vi "movimentacao basica.vi"() -> ()   [LabVIEW 2020]
uses:
  <vilib>/Utility/inputDevices.llb/joystickAcquire.vi
  <vilib>/Utility/inputDevices.llb/closeJoystick.vi
panel:
  out "Motor Esquerda":dbl
  out "Motor Direita":dbl
  out "Acelerando Trás":bool
  out "Acelerando Frente":bool
  out "Trás":bool
  out "Frente":bool
  out "joystick info":T1(array[cluster])
  out "axis info":T2
  out "button info":T3
  out "direction info":T4
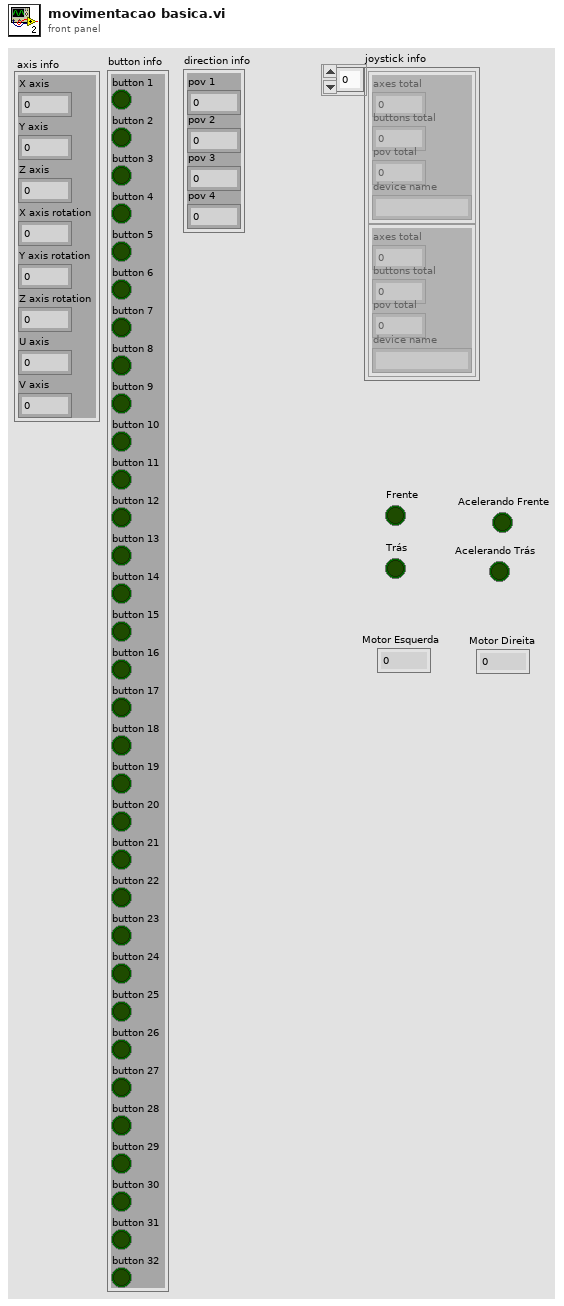
[diagram p1: front panel]
types:
  T1 = cluster{"axes total":u32, "buttons total":u32, "pov total":u32, "device name":string}[]
  T2 = cluster{"X axis":i32, "Y axis":i32, "Z axis":i32, "X axis rotation":i32, "Y axis rotation":i32, "Z axis rotation":i32, "U axis":i32, "V axis":i32}
  T3 = cluster{"button 1":bool, "button 2":bool, "button 3":bool, "button 4":bool, "button 5":bool, "button 6":bool, "button 7":bool, "button 8":bool, "button 9":bool, "button 10":bool, "button 11":bool, "button 12":bool, "button 13":bool, "button 14":bool, "button 15":bool, "button 16":bool, "button 17":bool, "button 18":bool, "button 19":bool, "button 20":bool, "button 21":bool, "button 22":bool, "button 23":bool, "button 24":bool, "button 25":bool, "button 26":bool, "button 27":bool, "button 28":bool, "button 29":bool, "button 30":bool, "button 31":bool, "button 32":bool}
  T4 = cluster{"pov 1":i32, "pov 2":i32, "pov 3":i32, "pov 4":i32}
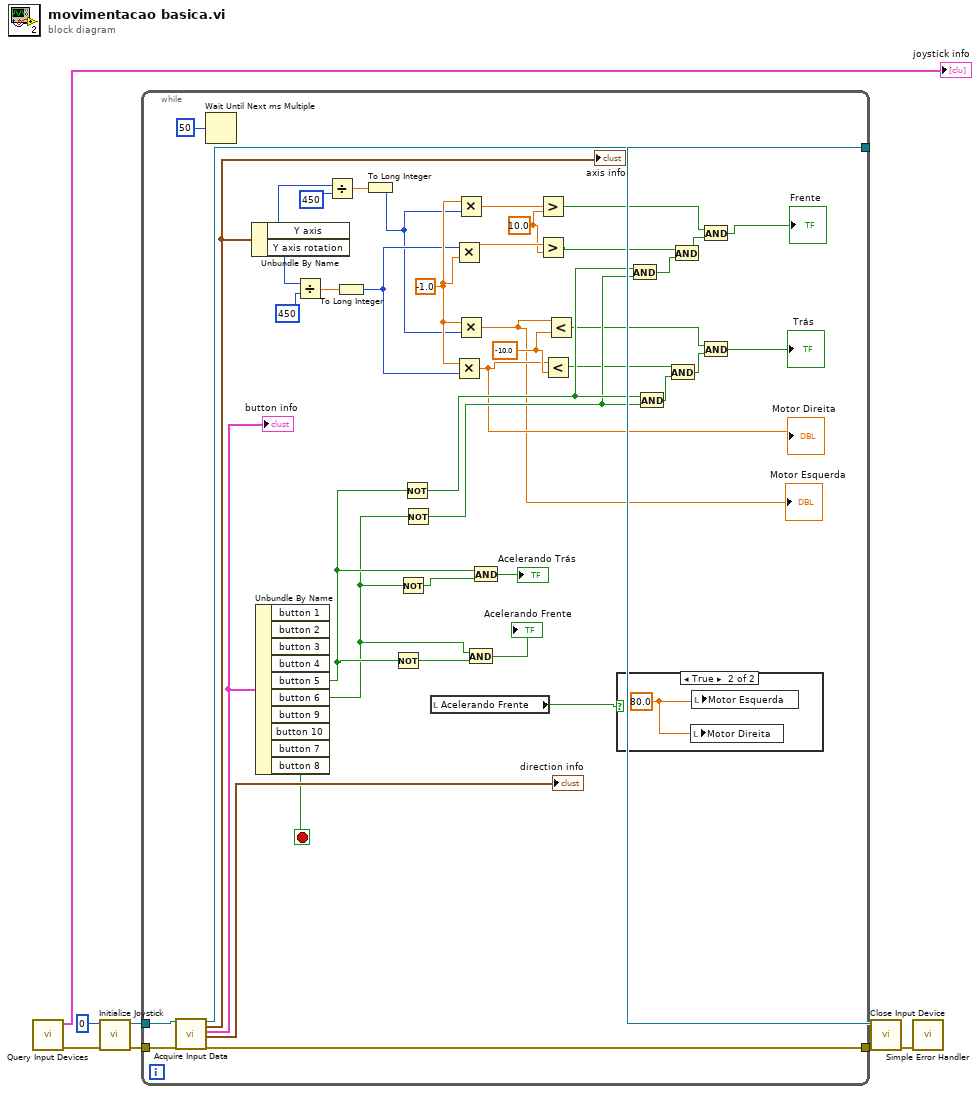
[diagram p0: block diagram]
diagram:
  n1 = call <vilib>:"Query Input Devices.vi"() -> ("error out"=w2:errorcluster, "joystick info"=→"joystick info":T1)  [unwired: 1 in, 9 out]
  n2 = call <vilib>:"Initialize Joystick.vi"("error in (no error)"=w2, "device index"=0) -> ("error out"=w6:errorcluster, "device ID"=w7:refnum<k1>)  [unwired: 8 out]
  n3 = while {
    tunnel: w7 -> [w51]
    tunnel: w6 -> [w50]
    tunnel: [w49] -> w5
    tunnel: [w46] -> w4
    stop <- w44 stop-if-true
    w19 = 10.0 ("y")
    w22 = -10.0 ("y")
    w42 = -1.0 ("x")
    n4 = call-poly <vilib>:"Acquire Input Data.vi"("device ID"=w51, "error in (no error)"=w50) -> ("device ID"=w49:refnum<k1>, "axis info"=w47:T2, "button info"=w40:T3, "direction info"=→"direction info":T4, "error out"=w46:errorcluster)  [unwired: 13 out]
    "axis info" <- w47
    "button info" <- w40
    n5 = Wait Until Next ms Multiple(millisecond multiple=u32 50) -> ()  [unwired: 1 out]
    n6 = Unbundle By Name(w47) -> ("Y axis"=w20:i32, "Y axis rotation"=w17:i32)
    n7 = Unbundle By Name(w40) -> ("button 5"=w29:bool, "button 6"=w28:bool, "button 7"=w44:bool)  [unwired: 7 out]
    n8 = Divide(x=w17, y=450) -> (x/y=w12:dbl)
    n9 = Divide(x=w20, y=450) -> (x/y=w11:dbl)
    n10 = To Long Integer(number=w12) -> (32bit integer=w13:i32)
    n11 = To Long Integer(number=w11) -> (32bit integer=w10:i32)
    n12 = Not(x=w29) -> (.not. x?=w30:bool)
    n13 = Not(x=w28) -> (.not. x?=w31:bool)
    n14 = Not(x=w29) -> (.not. x?=w34:bool)
    n15 = Not(x=w28) -> (.not. x?=w33:bool)
    n16 = local read "Acelerando Frente"() -> (w9:bool)
    n17 = Multiply(x=w13, y=w42) -> (x*y=w21:dbl)
    n18 = Multiply(x=w42, y=w13) -> (x*y=w15:dbl)
    "Motor Direita" <- w15
    n19 = Multiply(x=w42, y=w10) -> (x*y=w26:dbl)
    n20 = Multiply(x=w42, y=w10) -> (x*y=w14:dbl)
    "Motor Esquerda" <- w14
    n21 = And(x=w28, y=w30) -> (x .and. y?=→"Acelerando Frente":bool)
    n22 = And(x=w29, y=w31) -> (x .and. y?=→"Acelerando Trás":bool)
    n23 = Greater?(x=w26, y=w19) -> (0:w25:bool)
    n24 = Greater?(x=w21, y=w19) -> (0:w36:bool)
    n25 = Less?(x=w15, y=w22) -> (x < y?=w23:bool)
    n26 = Less?(x=w14, y=w22) -> (x < y?=w24:bool)
    n27 = case shown="True" w9 {
      frame False {
      }
      frame True {
        w52 = 80.0 ("Motor Esquerda")
        n28 = local write "Motor Direita"(w52) -> ()
        n29 = local write "Motor Esquerda"(w52) -> ()
      }
    }
    n30 = And(x=w34, y=w33) -> (x .and. y?=w35:bool)
    n31 = And(x=w34, y=w33) -> (x .and. y?=w38:bool)
    n32 = And(x=w23, y=w38) -> (x .and. y?=w39:bool)
    n33 = And(x=w36, y=w35) -> (x .and. y?=w37:bool)
    n34 = And(x=w25, y=w37) -> (x .and. y?=→"Frente":bool)
    n35 = And(x=w24, y=w39) -> (x .and. y?=→"Trás":bool)
  }
  n36 = call-poly <vilib>:"Close Input Device.vi"("error in (no error)"=w4, "device ID"=w5) -> ("error out"=w1:errorcluster)  [unwired: 8 out]
  n37 = call <vilib>:"Simple Error Handler.vi"("error in (no error)"=w1) -> ()  [unwired: 1 in, 8 out]
